vi "AlliGator Get ROI Intensity Array v4.vi"(8 "error in (no error)":errorcluster, 10 "ROI Descriptor":T2 {"Contours"."Type" items=["No Selection", "Point", "Line", "Rectangle", "Oval", "Polygon", "Freehand Region", "Annulus", "Unused2", "Unused3", "Broken Line", "Freehand Line", "Rotated Rectangle"]}, 11 "Images":cluster{"Image Sum":T1, "Image Array":T1[]}) -> (0 "Error Out":errorcluster, 1 "# Valid Pixels":i32, 2 "# Pixels":i32, 3 "ROI Intensity Array":dbl[](array[numeric]), 4 "CPU (s)":dbl, 5 "ROI Center":cluster{"X":i32, "Y":i32})   [LabVIEW 2021, in "AlliGator Decay Analysis.lvlib" / "AlliGator Decay Processing.lvlib"]
doc: "Gets the intensity array for the provided ROI."
uses:
  AlliGator Decay Processing.lvlib
  <vilib>/vision/Image Controls.llb/IMAQ Image.ctl
  AlliGator Source Image.lvlib
  Time/Time.lvlib
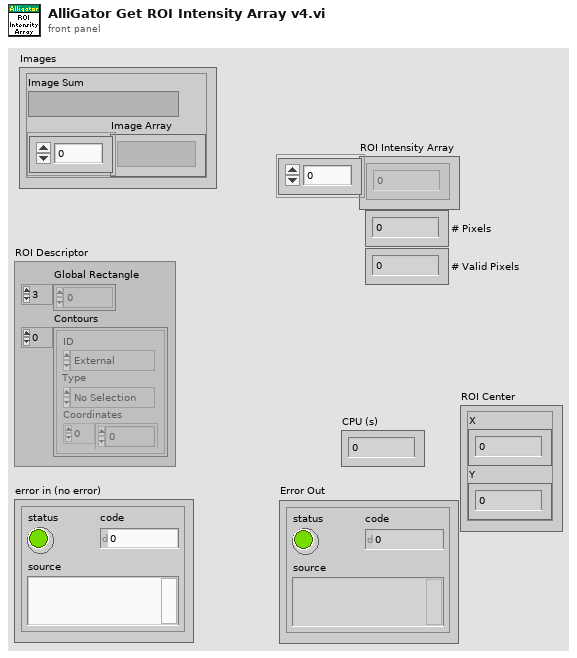
[diagram p1: front panel]
types:
  T1 = typedef "IMAQ Image.ctl" = refnum<image>
  T2 = typedef "ROI Descriptor" = cluster{"Global Rectangle":i32[], "Contours":cluster{"ID":enum32{"External", "Internal"}, "Type":u32, "Coordinates":i32[]}[]}
  T3 = typedef "AlliGator Settings.lvlib/AlliGator Pixel Counts Constraints.ctl" = cluster{"High Count Pixels Rejection Options":T4, "Low Count Pixels Rejection Options":T5}
  T4 = typedef "AlliGator Settings.lvlib/AlliGator High Count Pixels Rejection Options.ctl" = cluster{"Background High Threshold Factor":dbl, "Fixed High Background Threshold":dbl, "Reject High Count Pixels":bool, "High Percentile":dbl}
  T5 = typedef "AlliGator Settings.lvlib/AlliGator Low Count Pixels Rejection Options.ctl" = cluster{"Background Low Threshold Factor":dbl, "Fixed Low Background Threshold":dbl, "Reject Low Count Pixels":bool, "Low Percentile":dbl}
  T6 = cluster{"Decay Peak Constraint":bool, "Min":dbl, "Max":dbl}
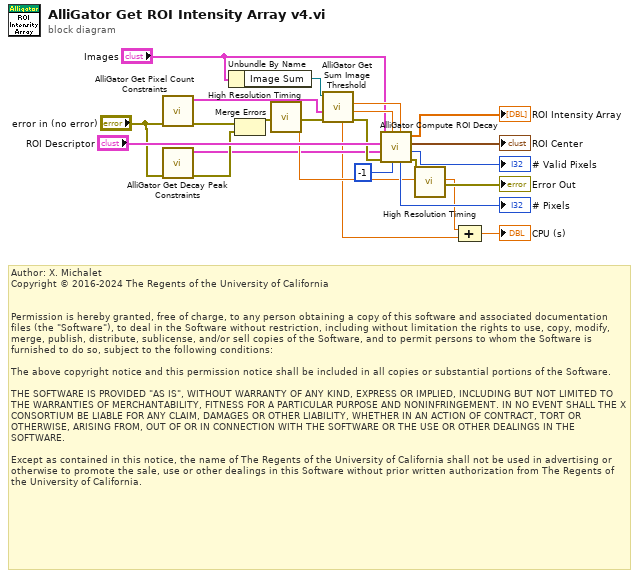
[diagram p0: block diagram]
diagram:
  # "Author: X. Michalet\nCopyright © 2016-2024 The Regents of the University of California\n \n\nPermission is hereby granted, free of charge, to any person obtaining a copy of this software and associated documentation files (the \"Software\"), to deal in the Software without restriction, including without limitation the rights to use, copy, modify, merge, publish, distribute, sublicense, and/or sell copies of the Software, and to permit persons to whom the Software is furnished to do so, subject to the following conditions:\n\nThe above copyright notice and this permission notice shall be included in all copies or substantial portions of the Software.\n\nTHE SOFTWARE IS PROVIDED \"AS IS\", WITHOUT WARRANTY OF ANY KIND, EXPRESS OR IMPLIED, INCLUDING BUT NOT LIMITED TO THE WARRANTIES OF MERCHANTABILITY, FITNESS FOR A PARTICULAR PURPOSE AND NONINFRINGEMENT. IN NO EVENT SHALL THE X CONSORTIUM BE LIABLE FOR ANY CLAIM, DAMAGES OR OTHER LIABILITY, WHETHER IN AN ACTION OF CONTRACT, TORT OR OTHERWISE, ARISING FROM, OUT OF OR IN CONNECTION WITH THE SOFTWARE OR THE USE OR OTHER DEALINGS IN THE SOFTWARE.\n\nExcept as contained in this notice, the name of The Regents of the University of California shall not be used in advertising or otherwise to promote the sale, use or other dealings in this Software without prior written authorization from The Regents of the University of California."
  n1 = call "AlliGator Get Pixel Count Constraints.vi"("error in (no error)"="error in (no error)") -> ("error out"=w24:errorcluster, "Pixel Count Constraints"=w4:T3)  [unwired: 9 in]
  n2 = call "AlliGator Get Decay Peak Constraints.vi"("error in (no error)"="error in (no error)") -> ("Error Out"=w11:errorcluster, "Decay Peak Constraints"=w5:T6)  [unwired: 9 in]
  n3 = Unbundle By Name("Images") -> ("Image Sum"=w21:T1)
  n4 = Merge Errors(w24, w11) -> (w23:errorcluster)
  n5 = call "High Resolution Timing.vi"("Error In"=w23) -> ("elapsed (relative) seconds"=w7:dbl, "Error Out"=w9:errorcluster)  [unwired: 16 in, 1 out]
  n6 = call "AlliGator Get Sum Image Threshold.vi"("error in (no error)"=w9, "Pixel Counts Constraints"=w4, "Image in"=w21) -> ("error out"=w12:errorcluster, "Pixel Threshold Low"=w14:sgl, "Pixel Threshold High"=w15:sgl, "elapsed (relative) seconds"=w2:dbl)  [unwired: 2 in, 3 out]
  n7 = call "AlliGator Compute ROI Decay.vi"("Pixel Threshold High"=w15, "Loop ID"=-1, "Pixel Threshold Low"=w14, "error in (no error)"=w12, "Decay Peak  Constraints"=w5, "ROI Descriptor"="ROI Descriptor", "Images"="Images") -> ("error out"=w22:errorcluster, "# Valid Pixels"=→"# Valid Pixels":i32, "ROI Center"=→"ROI Center":cluster{"X":i32, "Y":i32}, "Decay Points"=→"ROI Intensity Array":dbl[], "# Pixels"=→"# Pixels":i32)
  n8 = call "High Resolution Timing.vi"("relative seconds (NaN)"=w7, "Error In"=w22) -> ("elapsed (relative) seconds"=w6:dbl, "Error Out"=→"Error Out":errorcluster)  [unwired: 15 in, 1 out]
  n9 = Compound Arithmetic op=ADD(w6, w2) -> (→"CPU (s)":dbl)
